vi "WaitForMouseclick.vi"(2 "index In":i32, 3 "Origin":cluster{"left":i16, "top":i16}) -> (0 "index":i32, 1 "Dest":cluster{"left":i16, "top":i16})   [LabVIEW 2012]
panel:
  out "timed out?":bool
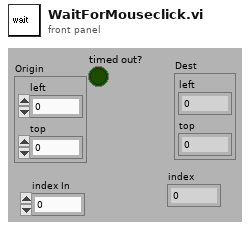
[diagram p1: front panel]
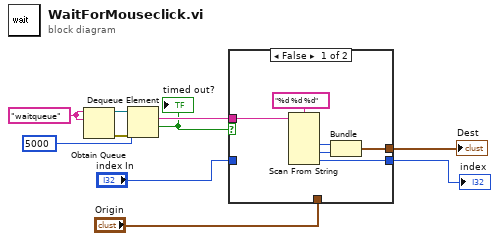
[diagram p0: block diagram]
diagram:
  w5 = "waitqueue" ("name (unnamed)")
  n1 = Obtain Queue(name (unnamed)=w5, element data type=w5) -> (queue out=w6:refnum<queue>, error out=w7:errorcluster)  [unwired: 3 in, 1 out]
  n2 = Dequeue Element(queue=w6, timeout in ms (-1)=5000, error in (no error)=w7) -> (element=w8:string, timed out?=w4:bool)  [unwired: 2 out]
  "timed out?" <- w4
  n3 = case shown="False" w4 {
    tunnel: [w16 w17] -> w9
    tunnel: w8 -> [w14 _]
    tunnel: [w11 w18] -> w1
    tunnel: "Origin" -> [_ w18]
    tunnel: "index In" -> [_ w17]
    frame False {
      n4 = Scan From String(format string="%d %d %d", input string=w14) -> (output 1=w13:i32, output 2=w12:i32, output 3=w16:i32)  [unwired: 5 in, 3 out]
      n5 = Bundle(w13, w12) -> (w11:cluster{i32, i32})  [unwired: 1 in]
    }
    frame True {
    }
  }
  "index" <- w9
  "Dest" <- w1
